vi "odch_std.vi"() -> ()   [LabVIEW 2025]
uses:
  <vilib>/Analysis/NI_AALBase.lvlib
panel:
  out "standard deviation":dbl format="%0.2f"
  out "odchylenie standardowe":dbl
  out "estymator nieobciazany wariancji":dbl
  out "Gaussian noise pattern":dbl[](array[numeric])
  in  "liczba cykli":i64
  in  "samples":i32=128
  in  "Sygnal":T1(ring)
  in  "phase":dbl
  in  "Amp":dbl
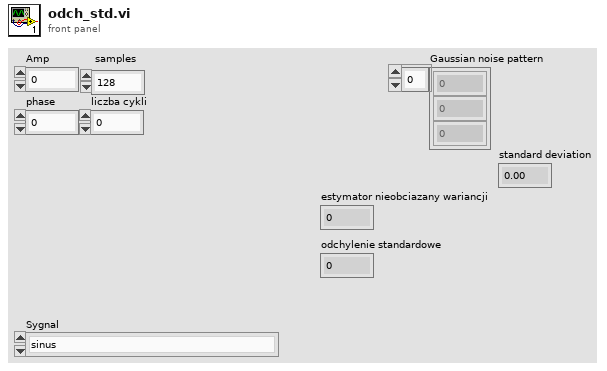
[diagram p1: front panel]
types:
  T1 = enum16{"sinus", "prostokat", "pila", "trojkat", "rozklad losowy", "rozklad normalny"}
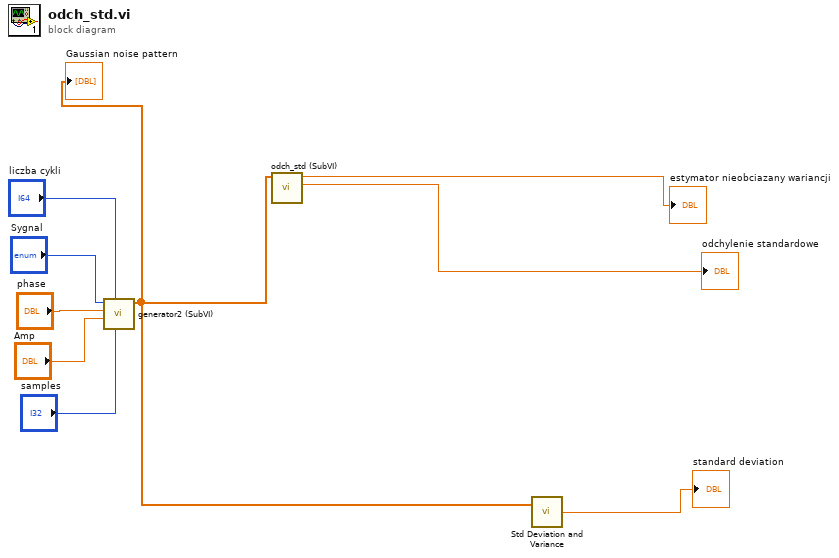
[diagram p0: block diagram]
diagram:
  n1 = call "generator2 (SubVI).vi"("samples"="samples", "liczba cykli"="liczba cykli", "Amp"="Amp", "phase"="phase", "Sygnal"="Sygnal") -> ("Gaussian noise pattern"=w3:dbl[])  [unwired: 6 in]
  "Gaussian noise pattern" <- w3
  n2 = call "odch_std (SubVI).vi"("Gaussian noise pattern"=w3) -> ("odchylenie standardowe"=→"odchylenie standardowe":dbl, "estymator nieobciazany wariancji"=→"estymator nieobciazany wariancji":dbl)  [unwired: 9 in]
  n3 = call <vilib>:"Std Deviation and Variance.vi"("X"=w3) -> ("standard deviation"=→"standard deviation":dbl)  [unwired: 1 in, 2 out]
